vi "ALTS-2015 LV2GBL DI status Info.vi"(7 "Options":T1, 8 "error in":errorcluster, 11 "DI Status":bool[](array[boolean])) -> (0 "error out":errorcluster, 3 "DI Status Out":bool[](array[boolean]))   [LabVIEW 2013]
uses:
  Controls/ALTS-2015 LV2GBL Options.ctl
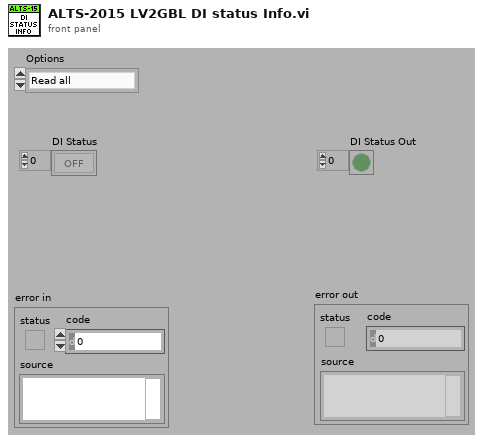
[diagram p1: front panel]
types:
  T1 = typedef "ALTS-2015 LV2GBL Options.ctl" = enum16{"Read all", "Write all"}
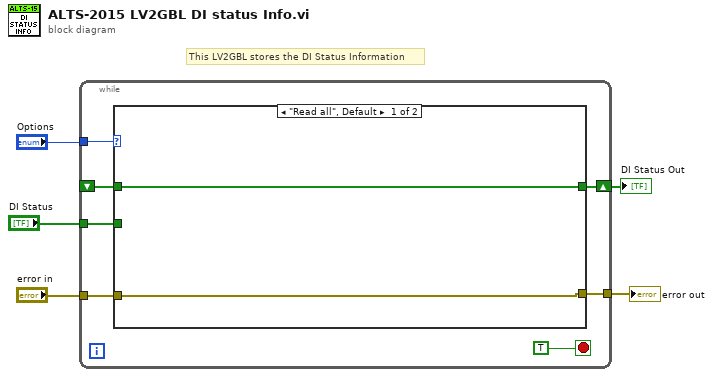
[diagram p0: block diagram]
diagram:
  # "This LV2GBL stores the DI Status Information"
  n1 = while {
    tunnel: "Options" -> [w11]
    tunnel: "error in" -> [w10]
    tunnel: [w9] -> w3
    shift-right: [w7] -> w1
    shift-left: _ -> [w8]
    tunnel: "DI Status" -> [w6]
    stop <- TRUE stop-if-true
    n2 = case shown="\"Read all\", Default" w11 {
      tunnel: [w14 w16] -> w9
      tunnel: w10 -> [w14 w16]
      tunnel: w8 -> [w13 _]
      tunnel: [w13 w15] -> w7
      tunnel: w6 -> [_ w15]
      frame "Read all", Default {
      }
      frame "Write all" {
      }
    }
  }
  "error out" <- w3
  "DI Status Out" <- w1
